vi "Method 3.vi"(10 "My Input":dbl, 11 "Test Actor 1 in":refnum<class "Test Async Actor.lvclass">) -> (2 "My Output":dbl, 3 "Test Actor 1 out":refnum<class "Test Async Actor.lvclass">)   [LabVIEW 2023, in "Test Async Actor.lvlib" / "Test Async Actor.lvclass"]
doc: "My Method Description"
uses:
  Test Async Actor.lvclass
  Test Async Actor.lvclass/Test Async Actor.ctl
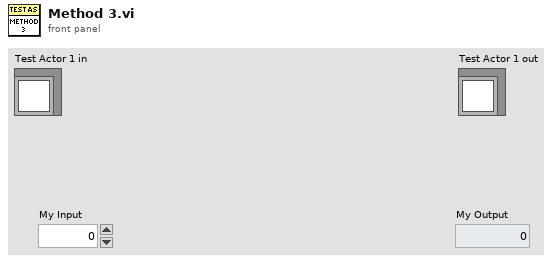
[diagram p1: front panel]
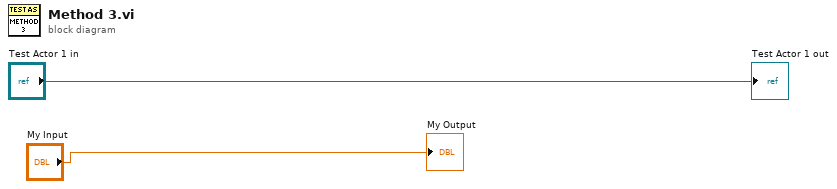
[diagram p0: block diagram]
diagram:
  "Test Actor 1 out" <- "Test Actor 1 in"
  "My Output" <- "My Input"
